vi "CheckFreeLibraryEntry.vi"(8 "ErrorIn":errorcluster caption="Error In(no Error)", 9 "LibraryName":string, 11 "ReferenceIn":refnum<class "ErrorDefinitionSQLite.lvclass"> caption="Reference In") -> (0 "ErrorOut":errorcluster caption="Error Out", 1 "FreeSpaceAvailable":bool, 3 "ReferenceOut":refnum<class "ErrorDefinitionSQLite.lvclass"> caption="Reference Out")   [LabVIEW 2021, in "ErrorDefinitionSQLite.lvclass"]
uses:
  ErrorDefinitionSQLite.lvclass
panel:
  out "FreeErrorCode":i32
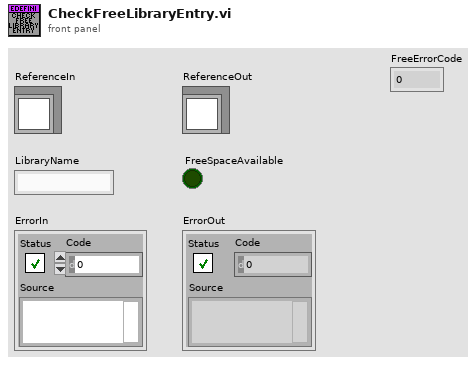
[diagram p1: front panel]
types:
  T1 = typedef "ErrorDefinitionSQLite.lvclass/ObjectAttributes.ctl" = cluster{"Path":path, "SQLiteRef":refnum<class "Connection.lvclass">, "EndOfRange":i32, "DefaultLibrarySize":i32, "StartOfRange":i32}
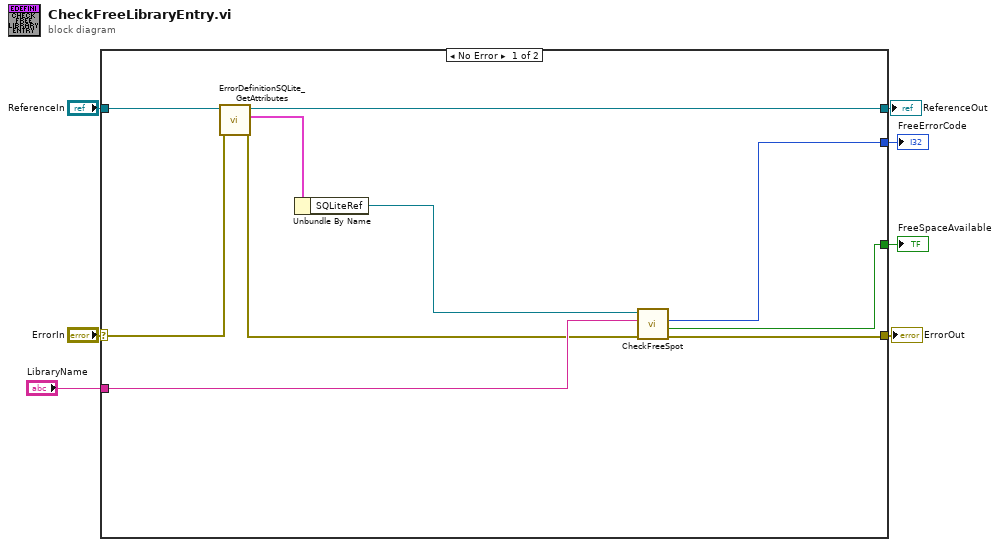
[diagram p0: block diagram]
diagram:
  n1 = case shown="No Error" "ErrorIn" {
    selector: "ErrorIn" -> [w17 w19]
    tunnel: [w12 w19] -> w6
    tunnel: [w15 w18] -> w4
    tunnel: "ReferenceIn" -> [w16 w18]
    tunnel: "LibraryName" -> [w13 _]
    tunnel: [w11 _] -> w2
    tunnel: [w10 _] -> w1
    frame No Error {
      n2 = call "ErrorDefinitionSQLite_GetAttributes.vi"("ErrorIn"=w17, "Reference in"=w16) -> ("ErrorOut"=w8:errorcluster, "Data"=w14:T1, "Reference out"=w15:refnum<class "ErrorDefinitionSQLite.lvclass">)  [unwired: 6 in, 1 out]
      n3 = Unbundle By Name(w14) -> ("SQLiteRef"=w9:refnum<class "Connection.lvclass">)
      n4 = call "CheckFreeSpot.vi"("error in (no error)"=w8, "LibraryName"=w13, "Connection in"=w9) -> ("error out"=w12:errorcluster, "Valid"=w11:bool, "ErrorCode"=w10:i32)  [unwired: 4 in, 2 out]
    }
    frame Error {
    }
  }
  "ErrorOut" <- w6
  "ReferenceOut" <- w4
  "FreeSpaceAvailable" <- w2
  "FreeErrorCode" <- w1
